vi "Name Label Opposite Visible Write.vi"(8 "error in (no error)":errorcluster, 9 "Caption Opposite Visible?":bool, 11 "3D Plot.lvclass in":refnum<class "3D Plot.lvclass">) -> (0 "error out":errorcluster, 3 "3D Plot.lvclass out":refnum<class "3D Plot.lvclass">)   [LabVIEW 2020, in "3D Plot.lvclass"]
uses:
  3D Plot.lvclass
  3D Plot.lvclass/3D Plot.ctl
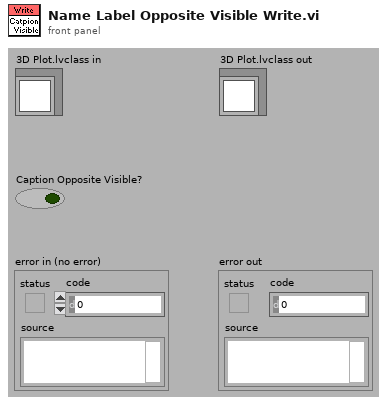
[diagram p1: front panel]
types:
  T1 = cluster{"Show Normal X Caption":bool, "Show Normal Y Caption":bool, "Show Normal Z Caption":bool, "Show Opposite X Caption":bool, "Show Opposite Y Caption":bool, "Show Opposite Z Caption":bool}
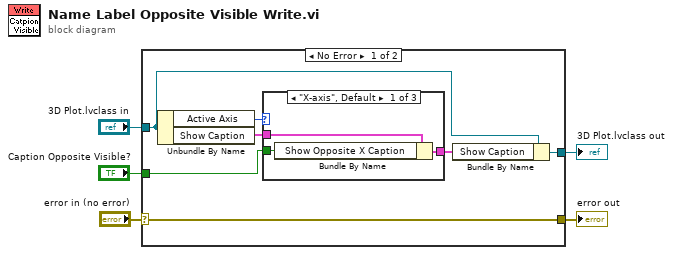
[diagram p0: block diagram]
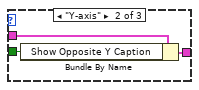
[diagram p2: hidden frame]
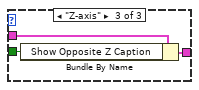
[diagram p3: hidden frame]
diagram:
  n1 = case shown="No Error" "error in (no error)" {
    selector: "error in (no error)" -> [w6 w22]
    tunnel: "Caption Opposite Visible?" -> [w12 _]
    tunnel: "3D Plot.lvclass in" -> [w8 w23]
    tunnel: [w7 w23] -> w3
    tunnel: [w6 w22] -> w1
    frame No Error {
      n2 = Unbundle By Name(w8) -> ("Active Axis"=w9:enum16{"X-axis", "Y-axis", "Z-axis"}, "Show Caption"=w10:T1)
      n3 = case shown="\"X-axis\", Default" w9 {
        tunnel: w10 -> [w15 w16 w20]
        tunnel: w12 -> [w14 w18 w21]
        tunnel: [w13 w17 w19] -> w11
        frame "X-axis", Default {
          n4 = Bundle By Name(cluster=w15, "Show Opposite X Caption"=w14) -> (w13:T1)
        }
        frame "Y-axis" {
          n5 = Bundle By Name(cluster=w16, "Show Opposite Y Caption"=w18) -> (w17:T1)
        }
        frame "Z-axis" {
          n6 = Bundle By Name(cluster=w20, "Show Opposite Z Caption"=w21) -> (w19:T1)
        }
      }
      n7 = Bundle By Name(cluster=w8, "Show Caption"=w11) -> (w7:refnum<class "3D Plot.lvclass">)
    }
    frame Error {
    }
  }
  "error out" <- w1
  "3D Plot.lvclass out" <- w3
